vi "readsettings.vi"() -> (0 "error out":errorcluster)   [LabVIEW 2012]
uses:
  globalsettings.vi
  <vilib>/Utility/config.llb/NI_LVConfig.lvlib
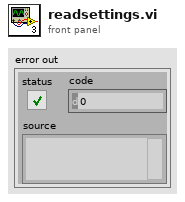
[diagram p1: front panel]
types:
  T1 = cluster{"DAC max":dbl, "DAC min":dbl, "DAC base":dbl, "DAC step":dbl, "Amplitude":dbl, "Tolerance":dbl, "Times":dbl}
  T2 = cluster{"Ten 0%":dbl, "Ten 5%":dbl, "Ten 10%":dbl, "Ten 15%":dbl, "Tolerance":dbl, "Ten 20%":dbl, "Ten 40%":dbl, "Ten 100%":dbl, "Times":dbl}
  T3 = cluster{"B0":dbl, "B1":dbl, "B2":dbl, "K":dbl, "B":dbl}
  T4 = cluster{"Ten 0%":dbl, "Ten 5%":dbl, "Ten 10%":dbl, "Ten 20%":dbl, "Tolerance":dbl, "Ten 15%":dbl, "Ten 40%":dbl, "Ten 100%":dbl, "Times":dbl}
  T5 = cluster{"B0":dbl, "B1":dbl, "K":dbl, "B":dbl, "B2":dbl}
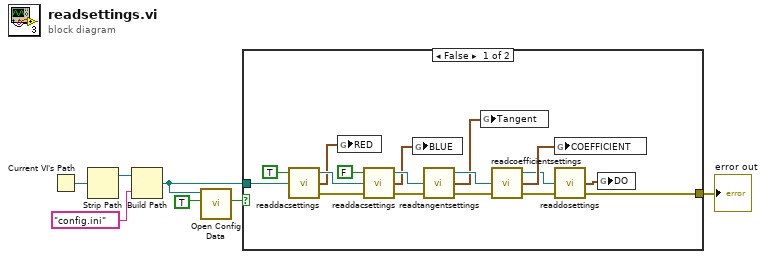
[diagram p0: block diagram]
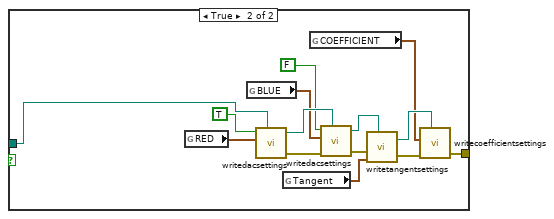
[diagram p2: hidden frame]
diagram:
  n1 = Current VI's Path() -> (path=w2:path)
  n2 = Strip Path(path=w2) -> (stripped path=w3:path)  [unwired: 1 out]
  n3 = Build Path(base path=w3, name or relative path="config.ini") -> (appended path=w4:path)
  n4 = call <vilib>:"Open Config Data.vi"("create file if necessary (T)"=TRUE, "configuration file path"=w4) -> ("file created?"=w5:bool)  [unwired: 7 in, 2 out]
  n5 = case shown="False" w5 {
    tunnel: w4 -> [w23 w38]
    tunnel: [w10 w25] -> w1
    frame False {
      n6 = call "readdacsettings.vi"("red"=TRUE, "Path"=w23) -> ("Path 2"=w22:path, 6:w18:T1, "error out"=w14:errorcluster)  [unwired: 3 in]
      n7 = global write "globalsettings.vi" "RED"(w18) -> ()
      n8 = call "readdacsettings.vi"("red"=FALSE, "Path"=w22, "error in (no error)"=w14) -> ("Path 2"=w19:path, 6:w17:T1, "error out"=w13:errorcluster)  [unwired: 2 in]
      n9 = global write "globalsettings.vi" "BLUE"(w17) -> ()
      n10 = call "readtangentsettings.vi"("Path"=w19, "error in (no error)"=w13) -> ("Path 2"=w20:path, 6:w16:T2, "error out"=w12:errorcluster)  [unwired: 3 in]
      n11 = global write "globalsettings.vi" "Tangent"(w16) -> ()
      n12 = call "readcoefficientsettings.vi"("Path"=w20, "error in (no error)"=w12) -> ("Path 2"=w9:path, 6:w15:T3, "error out"=w11:errorcluster)  [unwired: 3 in]
      n13 = global write "globalsettings.vi" "COEFFICIENT"(w15) -> ()
      n14 = call "readdosettings.vi"("Path"=w9, "error in (no error)"=w11) -> (6:w8:T2, "error out"=w10:errorcluster)  [unwired: 3 in, 1 out]
      n15 = global write "globalsettings.vi" "DO"(w8) -> ()
    }
    frame True {
      n16 = global read "globalsettings.vi" "RED"() -> (w29:T1)
      n17 = global read "globalsettings.vi" "BLUE"() -> (w30:T1)
      n18 = call "writedacsettings.vi"("red"=TRUE, "Path"=w38, 2:w29) -> ("Path 2"=w36:path, "error out"=w28:errorcluster)  [unwired: 4 in]
      n19 = global read "globalsettings.vi" "Tangent"() -> (w31:T4)
      n20 = global read "globalsettings.vi" "COEFFICIENT"() -> (w32:T5)
      n21 = call "writedacsettings.vi"("red"=FALSE, "Path"=w36, 2:w30, "error in (no error)"=w28) -> ("Path 2"=w34:path, "error out"=w27:errorcluster)  [unwired: 3 in]
      n22 = call "writetangentsettings.vi"("Path"=w34, 4:w31, "error in (no error)"=w27) -> ("error out"=w26:errorcluster, "Path 2"=w33:path)  [unwired: 3 in]
      n23 = call "writecoefficientsettings.vi"("Path"=w33, 2:w32, "error in (no error)"=w26) -> ("error out"=w25:errorcluster)  [unwired: 4 in, 1 out]
    }
  }
  "error out" <- w1
